vi "Fetal ECG Signal Extraction.vi"() -> ()   [LabVIEW 2023]
doc: "This example demonstrates how to extract fetal electrocardiogram (ECG) signals from maternal abdominal ECG signals. You obtain maternal abdominal ECG signals from obdominal leads. Maternal abdominal ECG signals contain both maternal ECG signals and fetal ECG signals. You can use an adaptive filter to extract fetal ECG signals from maternal abdominal ECG signals. To use an adaptive filter as the solution, you must obtain maternal thorax ECG signals from thorax leads as reference signals."
uses:
  <vilib>/addons/Adaptive Filters/Create/AFT Create FIR LMS (Real).vi
  <vilib>/addons/Adaptive Filters/Processing/AFT Filter Signal and Update Coefficients (Real, Waveform).vi
  <vilib>/addons/Adaptive Filters/NI_AdaptiveFilter.lvlib
panel:
  in  "Tab Control":enum32{"Background", "ECG Signals"}(tab)
  out "Maternal Abdominal ECG":waveform(dbl)(graph)
  out "Maternal Thorax ECG":waveform(dbl)(graph)
  out "Fetal ECG":waveform(dbl)(graph)
  in  "Step Size":dbl=0.45 min=0.0 step=0.01 format="%#_9f"
  in  "Filter Length":i32=40 min=2
  in  "Reference Signal: Maternal Thorax ECG":waveform(dbl)={"t0"=timestamp(0 s since 1904-01-01), "dt"=0.002, "Y"=array[5000 elements]}
  in  "Noisy Signal: Maternal Abdominal ECG":waveform(dbl)={"t0"=timestamp(0 s since 1904-01-01), "dt"=0.002, "Y"=array[5000 elements]}
  # "Fetal ECG signal extraction is one of adaptive noise cancellation applications. Refer to the Adaptive Noise Cancellation topic in the LabVIEW Help for more information about the background of adaptive noise cancellation. Select Help>>Show Context Help and move the cursor over the VI icon of this example for more information."
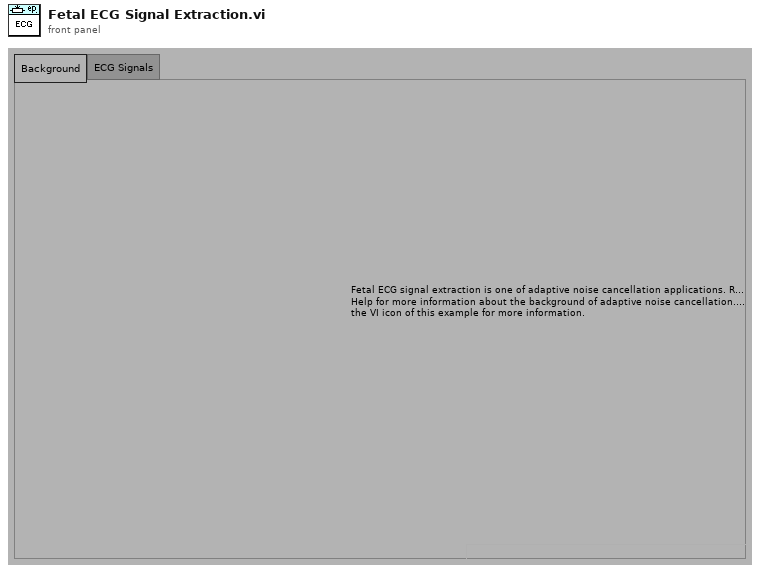
[diagram p1: front panel]
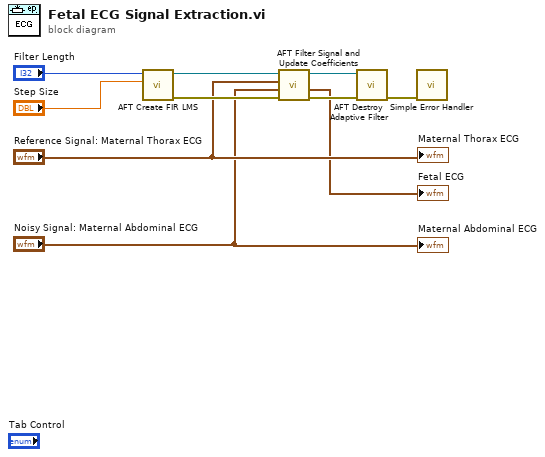
[diagram p0: block diagram]
diagram:
  n1 = call-poly <vilib>:"AFT Create FIR LMS.vi"("step size"="Step Size", "filter length"="Filter Length") -> ("error out"=w5:errorcluster, "adaptive filter out"=w6:refnum<k20>)  [unwired: 2 in, 6 out]
  n2 = call-poly <vilib>:"AFT Filter Signal and Update Coefficients.vi"("error in (no error)"=w5, "d(n)"="Noisy Signal: Maternal Abdominal ECG", "x(n)"="Reference Signal: Maternal Thorax ECG", "adaptive filter in"=w6) -> ("error out"=w9:errorcluster, "e(n)"=→"Fetal ECG":waveform(dbl), "adaptive filter out"=w10:refnum<k20>)  [unwired: 2 in, 3 out]
  n3 = call <vilib>:"AFT Destroy Adaptive Filter.vi"("error in (no error)"=w9, "adaptive filter in"=w10) -> ("error out"=w1:errorcluster)  [unwired: 9 out]
  n4 = call <vilib>:"Simple Error Handler.vi"("error in (no error)"=w1) -> ()  [unwired: 1 in, 8 out]
  "Maternal Thorax ECG" <- "Reference Signal: Maternal Thorax ECG"
  "Maternal Abdominal ECG" <- "Noisy Signal: Maternal Abdominal ECG"
